vi "Set Langauge (by VI).vi"(8 "error in":errorcluster, 9 "Target Language":string, 10 "VI Ref":refnum<vi>) -> (0 "error out":errorcluster)   [LabVIEW 2017, in "JKI Simple Localization.lvlib"]
doc: "Translates a single VI without adding it to the local registry.\n\nTarget Language: Optional input. Leave blank to use the default language."
uses:
  JKI Simple Localization.lvlib
  Definitions/Private/Translation.Action.ctl
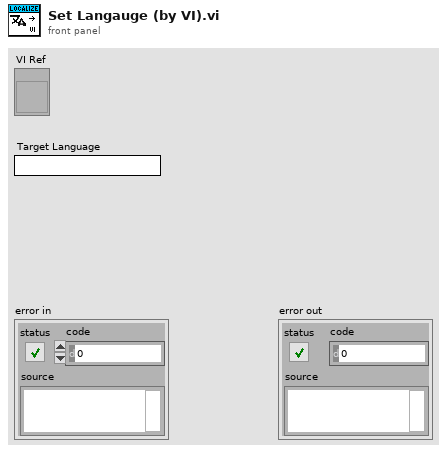
[diagram p1: front panel]
types:
  T1 = typedef "JKI Simple Localization.lvlib/Translation.Action.ctl" = enum16{"Read Dictionary", "Translate VIs", "Register VI", "Get Languages", "Translate Phrase", "Translate VI", "Unregister"}
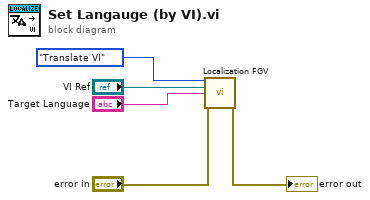
[diagram p0: block diagram]
diagram:
  n1 = call "Localization FGV.vi"("Action"=Translation.Action."Translate VI", "VI in"="VI Ref", "Target Language"="Target Language", "error in"="error in") -> ("error out"=→"error out":errorcluster)  [unwired: 7 in, 4 out]
